vi "总磷断电保存全局变量.vi"() -> ()   [LabVIEW 2016, in "斯坦道总磷.lvlib"]
panel:
  in  "MB通信方式选择":enum16{"串口", "TCP"}(ring)
  in  "PORT":string="502"
  in  "IP":string="192.168.1.204"
  in  "VISA Resource":refnum<visa-resource-name>="COM5"
  in  "运行周期":T1={"运行模式"=enum."维护模式", "质控频次"=enum."关闭", "空白核查时间"=2, "跨度核查时间"=6, "24H周期设置"=[]} {"跨度核查时间" items=["00H", "01H", "02H", "03H", "04H", "05H", "06H", "07H", "08H", "09H", "10H", "11H", "12H", "13H", "14H", "15H", "16H", "17H", "18H", "19H", "20H", "21H", "22H", "23H", "关闭"]; "空白核查时间" items=["00H", "01H", "02H", "03H", "04H", "05H", "06H", "07H", "08H", "09H", "10H", "11H", "12H", "13H", "14H", "15H", "16H", "17H", "18H", "19H", "20H", "21H", "22H", "23H", "关闭"]}
  in  "流程路径":path=path "C:/Users/std/Documents/斯坦道流程文件/流程.xml"
  in  "质控参数设置":T2
  in  "总磷自动测试量程配置":T3={"水样测试量程模式"=enum."AUTO", "空白核查量程模式"=enum."AUTO", "跨度核查量程模式"=enum."AUTO"}
  in  "定时控制":T4={"控制命令"=enum."启动测量", "周期设置类型"=enum."定点启动", "定时功能启用"=FALSE, "定时间隔"=1.0, "24H周期设置"=[], "零点核查时间"=2, "跨度核查时间"=6, "质控频次"=enum."关闭"} {"跨度核查时间" items=["00H", "01H", "02H", "03H", "04H", "05H", "06H", "07H", "08H", "09H", "10H", "11H", "12H", "13H", "14H", "15H", "16H", "17H", "18H", "19H", "20H", "21H", "22H", "23H", "关闭"]; "零点核查时间" items=["00H", "01H", "02H", "03H", "04H", "05H", "06H", "07H", "08H", "09H", "10H", "11H", "12H", "13H", "14H", "15H", "16H", "17H", "18H", "19H", "20H", "21H", "22H", "23H", "关闭"]}
  # "运行模式："
  # "质控频次："
  # "零点核查时间："
  # "跨度核查时间："
  # "质控参数设置"
  # "监测参数"
  # "总磷"
  # "跨度值"
  # "零点核查标准液浓度"
  # "跨度核查标准液浓度"
  # "标样核查标准液浓度"
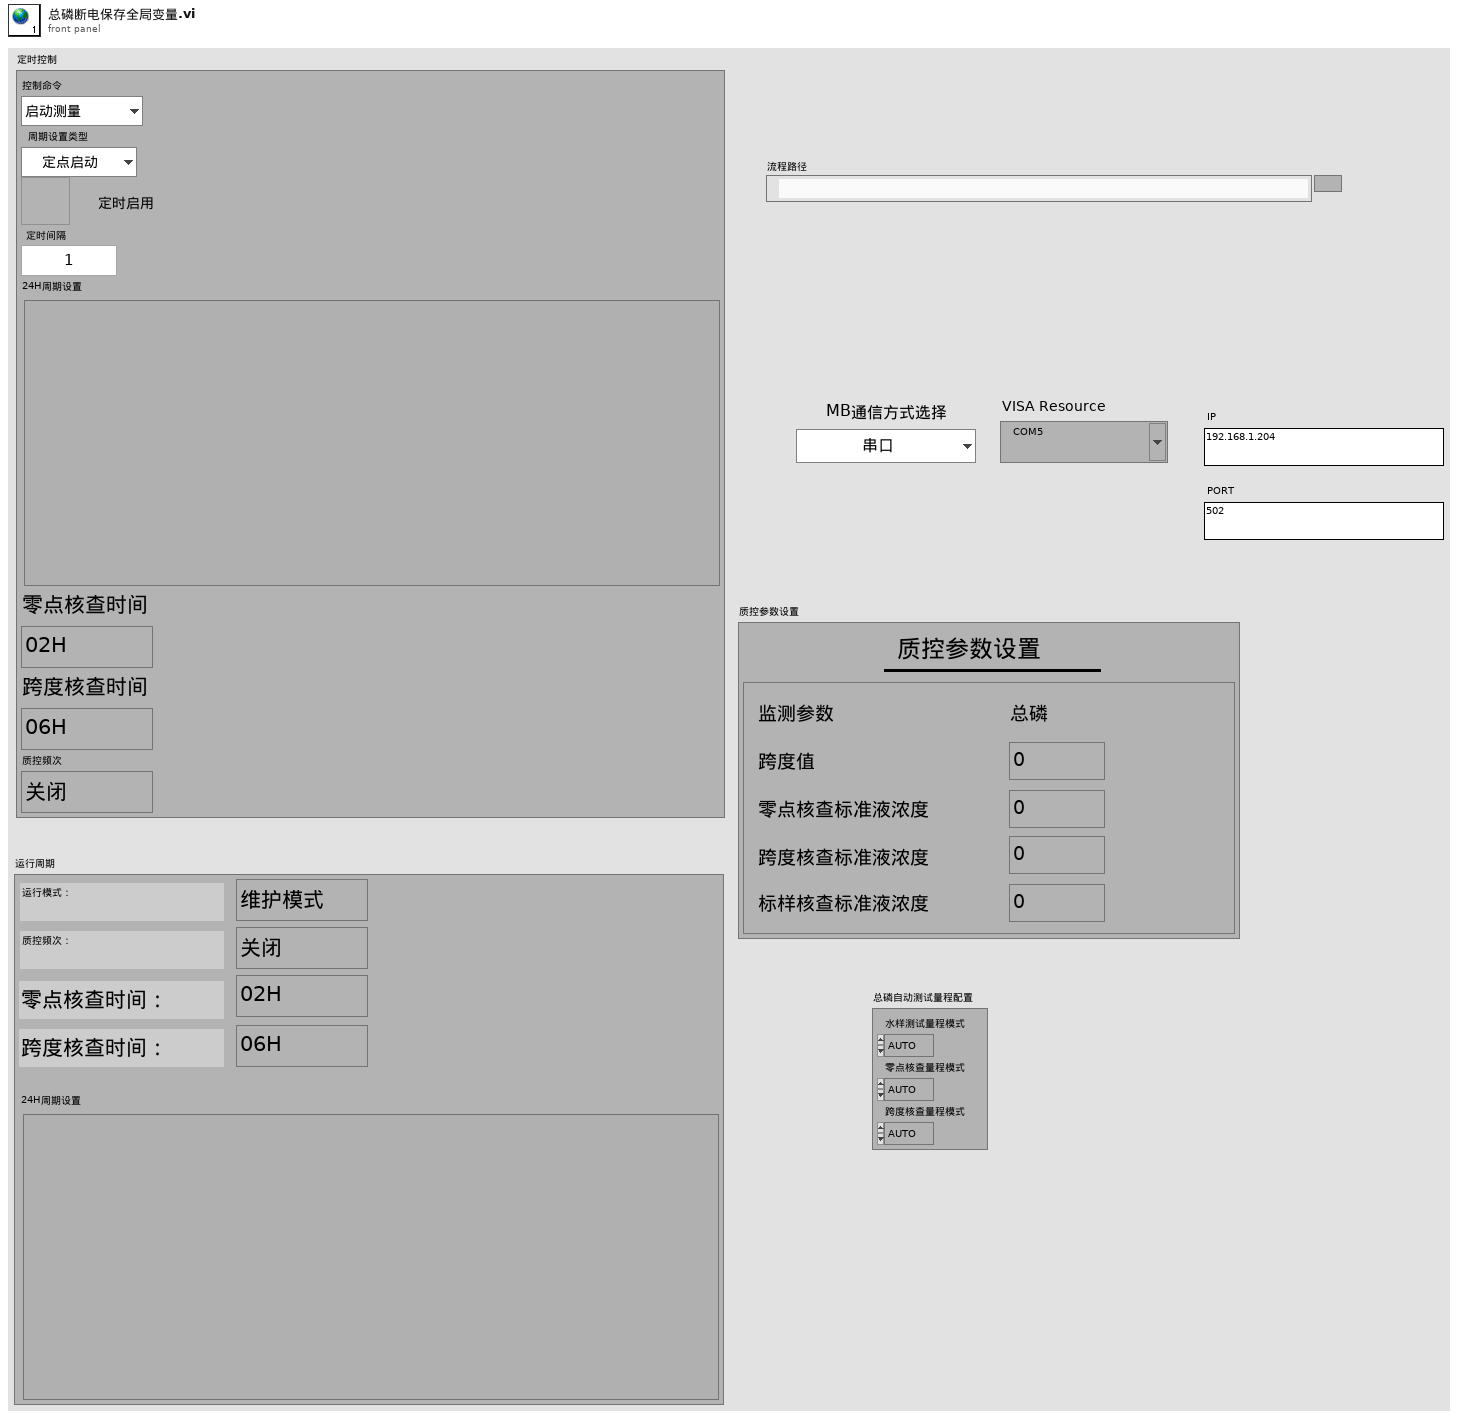
[diagram p1: front panel]
types:
  T1 = cluster{"运行模式":enum16{"维护模式", "常规模式", "应急模式", "质控模式"}, "质控频次":enum16{"关闭", "每天", "星期一", "星期二", "星期三", "星期四", "星期五", "星期六", "星期日"}, "空白核查时间":u16, "跨度核查时间":u16, "24H周期设置":bool[]}
  T2 = cluster{"总磷跨度值":dbl, "总磷零点标准液浓度":dbl, "总磷跨度标准液浓度":dbl, "总磷标准液标准浓度":dbl}
  T3 = cluster{"水样测试量程模式":enum16{"H", "L", "AUTO"}, "空白核查量程模式":enum16{"H", "L", "AUTO"}, "跨度核查量程模式":enum16{"H", "L", "AUTO"}}
  T4 = cluster{"控制命令":enum16{"启动测量", "标样核查", "零点核查", "跨度核查", "空白测试", "平行样测试", "加标回收", "空白校准", "标样校准", "初始化（清洗）", "停止测试", "仪器重启", "校时", "模式设置", "测量间隔设置"}, "周期设置类型":enum16{"定点启动", "间隔启动"}, "定时功能启用":bool, "定时间隔":dbl, "24H周期设置":bool[], "零点核查时间":u16, "跨度核查时间":u16, "质控频次":enum16{"关闭", "每天", "星期一", "星期二", "星期三", "星期四", "星期五", "星期六", "星期日"}}
diagram:
